vi "Pot Volts to Radians.vi"(1 "Volts In":dbl) -> (0 "Angle Delta Out":dbl)   [LabVIEW 2011]
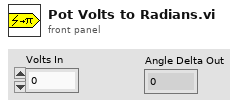
[diagram p1: front panel]
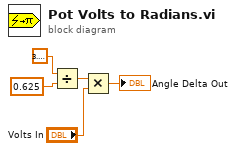
[diagram p0: block diagram]
diagram:
  n1 = Divide(x=3.141592653589793, y=0.625 ("x")) -> (x/y=w5:dbl)
  n2 = Multiply(x=w5, y="Volts In") -> (x*y=→"Angle Delta Out":dbl)
